vi "RC_Client N.vi"(8 "error in (no error)":errorcluster, 10 "#":i32, 11 "RC Type":T1) -> ()   [LabVIEW 2019, in "RemoteControl.lvlib" / "RemoteControl.lvclass"]
uses:
  RemoteControl.lvclass
  Typedefs/RC Com Type--enum.ctl
panel:
  # "CLIENT (API)"
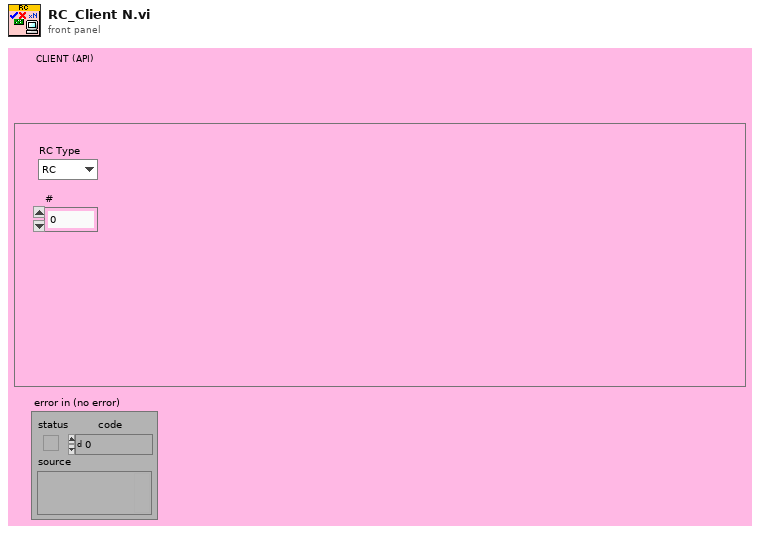
[diagram p1: front panel]
types:
  T1 = typedef "RemoteControl.lvlib/RemoteControl.lvclass/RC Com Type--enum.ctl" = enum16{"RC", "STM", "ZMQ"}
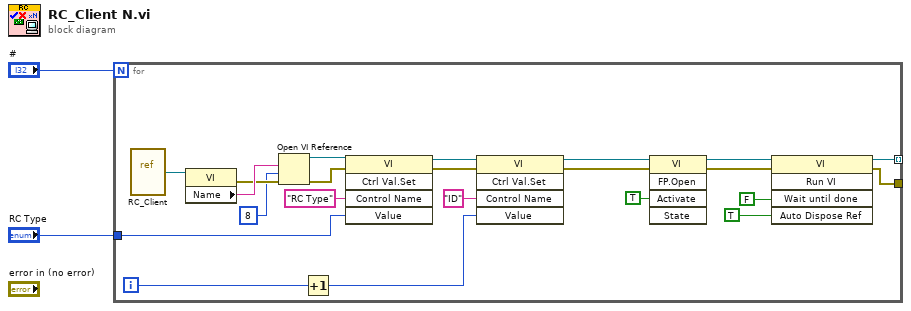
[diagram p0: block diagram]
diagram:
  n1 = for {
    N: "#" -> [_]
    tunnel: "RC Type" -> [w6]
    tunnel: [w5] -> _
    tunnel: [w4] -> _ mode=indexing
    i -> [w8]
    n2 = vi-ref "RC_Client.vi"() -> (w24:refnum<vi>)
    n3 = property class="VI"(reference=w24) -> (error out=w22:errorcluster, "Name"=w23:string)  [unwired: 1 in, 1 out]
    n4 = Open VI Reference(vi path=w23, options=8, error in (no error)=w22) -> (vi reference=w19:refnum<vi>, error out=w18:errorcluster)  [unwired: 3 in]
    n5 = Increment(x=w8) -> (x+1=w3:i32)
    n6 = invoke class="VI" method="Ctrl Val.Set"(reference=w19, error in=w18, "Control Name"="RC Type", "Value"=w6) -> (reference out=w16:refnum<vi>, error out=w15:errorcluster)  [unwired: 1 in, 3 out]
    n7 = invoke class="VI" method="Ctrl Val.Set"(reference=w16, error in=w15, "Control Name"="ID", "Value"=w3) -> (reference out=w13:refnum<vi>, error out=w12:errorcluster)  [unwired: 1 in, 3 out]
    n8 = invoke class="VI" method="FP.Open"(reference=w13, error in=w12, "Activate"=TRUE ("Activate?")) -> (reference out=w11:refnum<vi>, error out=w10:errorcluster)  [unwired: 2 in, 3 out]
    n9 = invoke class="VI" method="Run VI"(reference=w11, error in=w10, "Wait until done"=FALSE ("Wait Until Done"), "Auto Dispose Ref"=TRUE ("Auto Dispose Reference")) -> (reference out=w4:refnum<vi>, error out=w5:errorcluster)  [unwired: 1 in, 3 out]
  }
